vi "Create_Drive_Train_Base.vi"(10 "RobotDriveDevRef":T4={"DevStatus"={"status"=FALSE, "code"=0, "source"=""}, "Motors[]"=[], "Square Inputs"=FALSE, "Max Output"=1.0}, 11 "Drive Train":T9=enum."Tank Drive 4 Motor") -> (3 "DriveClusterOut":T1={"Sensor Data"={"Gyro Data"={"Gyro RT FIFO"=refnum, "Gyro Current"=0.0, "Gyro Hold"=0.0}, "Encoder Data"={"Encoder RT FIFO"=refnum, "Encoder Current"=0.0, "Encoder Hold"=0.0}, "Camera Data"={"Camera RT FIFO"=refnum, "Camera Current"={" Angle"=0.0, "Valid"=FALSE}}}, "RobotDriveDevRef"={"DevStatus"={"status"=FALSE, "code"=0, "source"=""}, "Motors[]"=[], "Square Inputs"=FALSE, "Max Output"=1.0}, "Drive Train"=enum."Tank Drive 2 Motor", "Valid Commands"=[], "Drive Comand Notifier"=refnum, "Command Finished?"=refnum, "Command Canceled"=refnum})   [LabVIEW 2016]
uses:
  <userlib>/836-libraries/Drive/Drive_Code_V2/Drive_Code_Support/DriveTrains/Drive_Trains.ctl
  <vilib>/Rock Robotics/WPI/RobotDrive/WPI_RobotDriveDevRef.ctl
  <vilib>/Rock Robotics/WPI/MotorControl/WPI_MotorControlDeviceRef.ctl
  <vilib>/Rock Robotics/WPI/MotorControl/WPI_MotorControlType.ctl
  <vilib>/Rock Robotics/SystemInterfaces/DIO/FPGA_DIOPWMChannel.ctl
  <vilib>/Rock Robotics/WPI/PWM/WPI_PWMDeadband.ctl
  <userlib>/836-libraries/Drive/Drive_Code_V2/Drive_Code_Support/Drive_Code_Bundle.ctl
  <userlib>/836-libraries/Drive/Drive_Code_V2/Drive_Code_Support/SensorTypedefs/Sensor_Cluster.ctl
  <userlib>/836-libraries/Drive/Drive_Code_V2/Drive_Code_Support/SensorTypedefs/Camera_Cluster.ctl
  <userlib>/836-libraries/Drive/Drive_Code_V2/Drive_Code_Support/Command_Sends/Drive_Code_Command_Type.ctl
  <userlib>/836-libraries/Drive/Drive_Code_V2/Drive_Code_Support/Command_Sends/Drive_Code_Command_List.ctl
  <vilib>/Rock Robotics/WPI/SafetyOutput/WPI_SafetyOutputConfigMenu.ctl
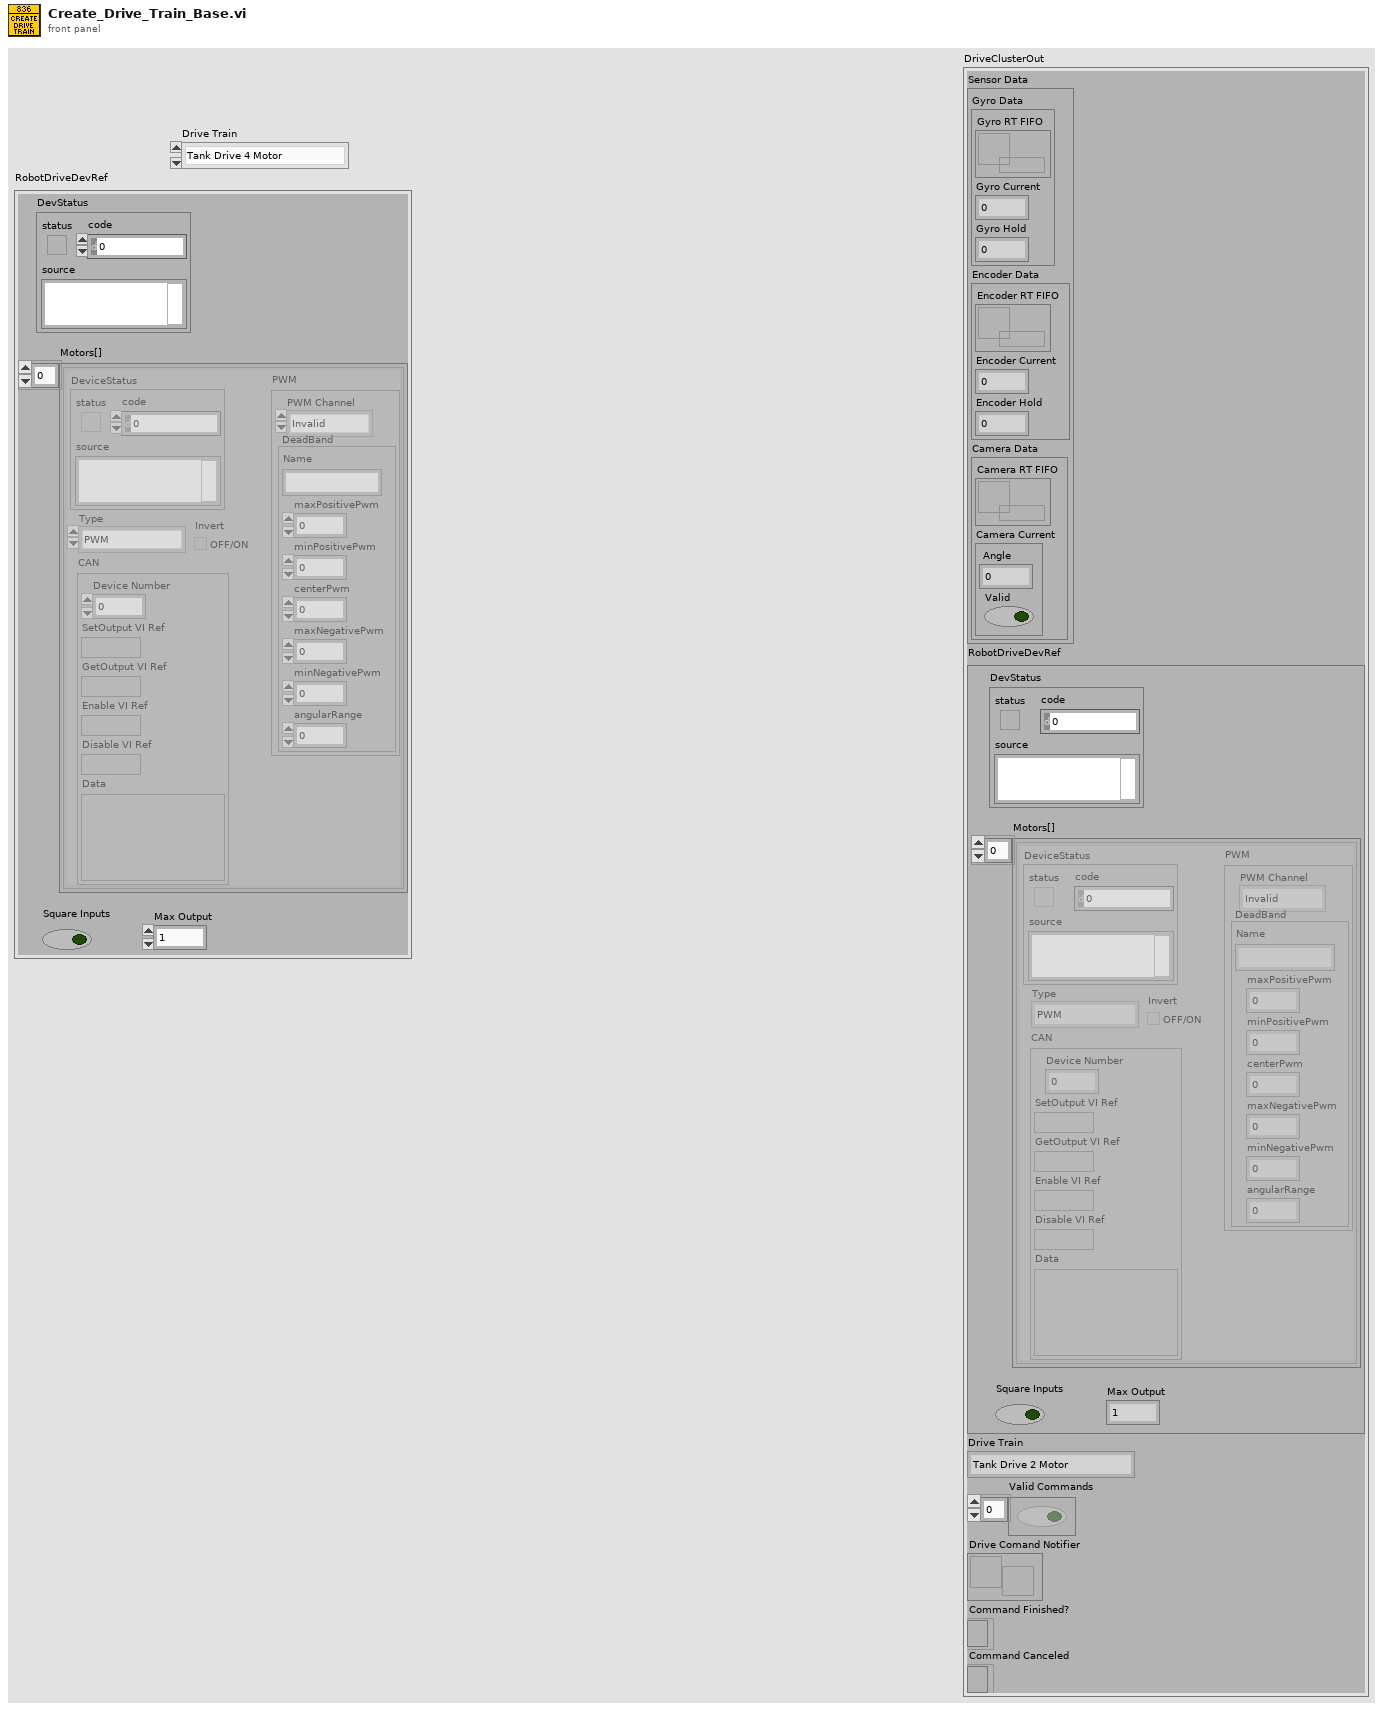
[diagram p1: front panel]
types:
  T1 = typedef "Drive_Code_Bundle.ctl" = cluster{"Sensor Data":T2, "RobotDriveDevRef":T4, "Drive Train":T9, "Valid Commands":bool[], "Drive Comand Notifier":refnum<notifier>, "Command Finished?":refnum<k4>, "Command Canceled":refnum<k4>}
  T2 = typedef "Sensor_Cluster.ctl" = cluster{"Gyro Data":cluster{"Gyro RT FIFO":refnum<k33>, "Gyro Current":dbl, "Gyro Hold":dbl}, "Encoder Data":cluster{"Encoder RT FIFO":refnum<k33>, "Encoder Current":dbl, "Encoder Hold":dbl}, "Camera Data":cluster{"Camera RT FIFO":refnum<k33>, "Camera Current":T3}}
  T3 = typedef "Camera_Cluster.ctl" = cluster{" Angle":dbl, "Valid":bool}
  T4 = typedef "WPI_RobotDriveDevRef.ctl" = cluster{"DevStatus":errorcluster, "Motors[]":T5[], "Square Inputs":bool, "Max Output":dbl}
  T5 = typedef "WPI_MotorControlDeviceRef.ctl" = cluster{"DeviceStatus":errorcluster, "Type":T6, "PWM":cluster{"PWM Channel":T7, "DeadBand":T8}, "CAN":cluster{"Device Number":u8, "SetOutput VI Ref":variant, "GetOutput VI Ref":variant, "Enable VI Ref":variant, "Disable VI Ref":variant, "Data":variant}, "Invert":bool}
  T6 = typedef "WPI_MotorControlType.ctl" = enum16{"PWM", "CAN"}
  T7 = typedef "FPGA_DIOPWMChannel.ctl" = enum8{"PWM 0", "PWM 1", "PWM 2", "PWM 3", "PWM 4", "PWM 5", "PWM 6", "PWM 7", "PWM 8", "PWM 9", "PWM MXP 0", "PWM MXP 1", "PWM MXP 2", "PWM MXP 3", "PWM MXP 4", "PWM MXP 5", "PWM MXP 6", "PWM MXP 7", "PWM MXP 8", "PWM MXP 9", "Invalid"}
  T8 = typedef "WPI_PWMDeadband.ctl" = cluster{"Name":string, "maxPositivePwm":i32, "minPositivePwm":i32, "centerPwm":i32, "maxNegativePwm":i32, "minNegativePwm":i32, "angularRange":u16}
  T9 = typedef "Drive_Trains.ctl" = enum16{"Tank Drive 2 Motor", "Tank Drive 4 Motor", "Mecanum Drive", "Kiwi Drive"}
  T10 = typedef "WPI_SafetyOutputConfigMenu.ctl" = enum16{"Enable", "Disable"}
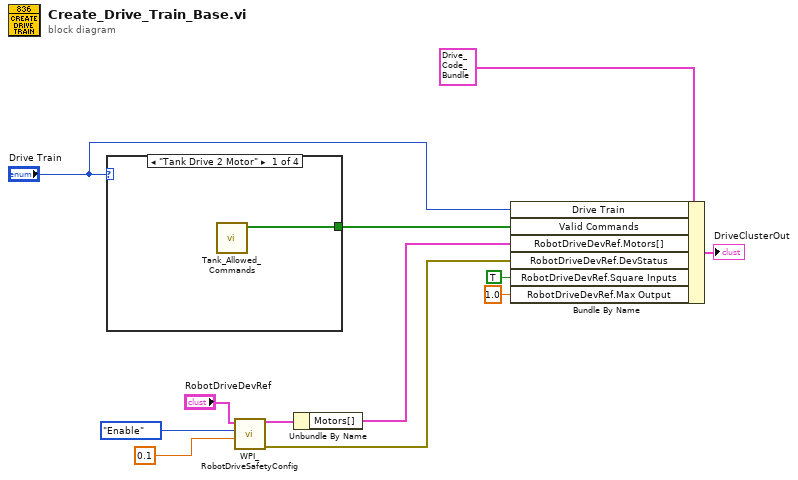
[diagram p0: block diagram]
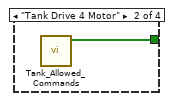
[diagram p2: hidden frame]
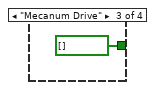
[diagram p3: hidden frame]
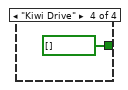
[diagram p4: hidden frame]
diagram:
  n1 = case shown="\"Tank Drive 2 Motor\"" "Drive Train" {
    tunnel: [w13 w14 bool[] [] ("Array") bool[] [] ("Array")] -> w3
    frame "Tank Drive 2 Motor" {
      n2 = call <userlib>:"Tank_Allowed_Commands.vi"() -> ("Array"=w13:bool[])  [unwired: 11 in]
    }
    frame "Tank Drive 4 Motor" {
      n3 = call <userlib>:"Tank_Allowed_Commands.vi"() -> ("Array"=w14:bool[])  [unwired: 11 in]
    }
    frame "Mecanum Drive" {
    }
    frame "Kiwi Drive" {
    }
  }
  n4 = call <vilib>:"WPI_RobotDriveSafetyConfig.vi"("timeout (s)"=0.1, "mode"=WPI_SafetyOutputConfigMenu."Enable", "RobotDriveDevRef"="RobotDriveDevRef") -> ("error out"=w6:errorcluster, "RobotDriveDevRef"=w5:T4)  [unwired: 7 in]
  n5 = Unbundle By Name(w5) -> ("Motors[]"=w4:T5[])
  n6 = Bundle By Name(cluster=T1 {"Sensor Data"={"Gyro Data"={"Gyro RT FIFO"=refnum, "Gyro Current"=0.0, "Gyro Hold"=0.0}, "Encoder Data"={"Encoder RT FIFO"=refnum, "Encoder Current"=0.0, "Encoder Hold"=0.0}, "Camera Data"={"Camera RT FIFO"=refnum, "Camera Current"={" Angle"=0.0, "Valid"=FALSE}}}, "RobotDriveDevRef"={"DevStatus"={"status"=FALSE, "code"=0, "source"=""}, "Motors[]"=[], "Square Inputs"=FALSE, "Max Output"=1.0}, "Drive Train"=enum."Tank Drive 4 Motor", "Valid Commands"=[], "Drive Comand Notifier"=refnum, "Command Finished?"=refnum, "Command Canceled"=refnum} ("Cluster"), "Drive Train"="Drive Train", "Valid Commands"=w3, "RobotDriveDevRef.Motors[]"=w4, "RobotDriveDevRef.DevStatus"=w6, "RobotDriveDevRef.Square Inputs"=TRUE, "RobotDriveDevRef.Max Output"=1.0) -> (→"DriveClusterOut":T1)
